vi "sg Set ASK.vi"(0 "device":i32, 1 "depth":dbl, 2 "symbolCount":i32, 5 "symbolRate":dbl, 7 "filterType":u32(ring) items=["sgRaisedCosine", "sgRootRaisedCosine", "sgGaussian", "sgNone"], 9 "filterAlpha":dbl, 11 "error in (no error)":errorcluster, 12 "symbols":i32) -> (4 "function return":u32(ring), 14 "symbols out":i32, 15 "error out":errorcluster)   [LabVIEW 2014, in "VSG25A.lvlib"]
doc: "SG_API sgStatus sgSetASK(int device, double symbolRate, sgFilterType filterType,\n double filterAlpha, double depth, int *symbols, int symbolCount);"
uses:
  VSG25A.lvlib
  sg_api.dll
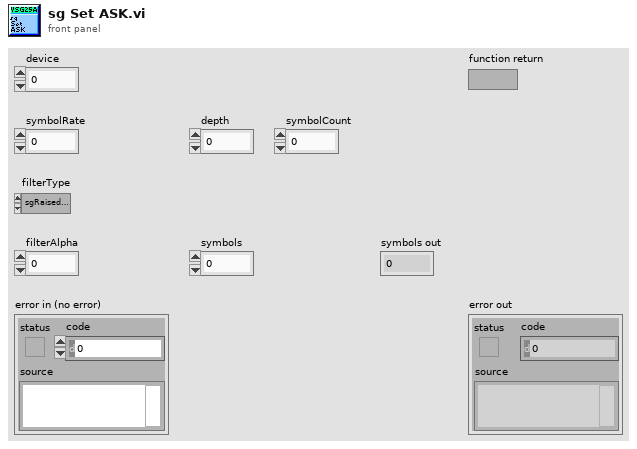
[diagram p1: front panel]
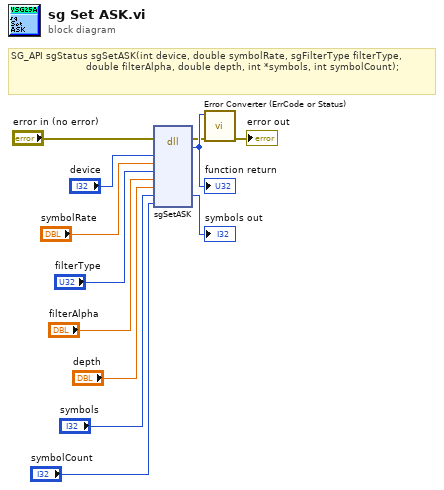
[diagram p0: block diagram]
diagram:
  # "SG_API sgStatus sgSetASK(int device, double symbolRate, sgFilterType filterType,\n                         double filterAlpha, double depth, int *symbols, int symbolCount);"
  n1 = dll-call lib="C:/Users/M_LAPTOP/Desktop/Labview/practice/VSG25A/sg_lib/sg_api.*" fn="sgSetASK"(error in="error in (no error)", "device"="device", "symbolRate"="symbolRate", "filterType"="filterType", "filterAlpha"="filterAlpha", "depth"="depth", "symbols"="symbols", "symbolCount"="symbolCount") -> (error out=w2:errorcluster, w12:u32, "symbols"=→"symbols out":i32)  [unwired: 8 in, 1 out]
  "function return" <- w12
  n2 = call "Error Converter (ErrCode or Status).vi"("error in (no error)"=w2, "error code"=w12) -> ("error out"=→"error out":errorcluster)  [unwired: 9 in]
